vi "Initialise Survey Polygons.vi"(0 "Camera Settings":T2, 5 "Altitude (m)":dbl, 7 "Overlap (%)":dbl, 11 "Error In":errorcluster) -> (2 "Points of Polygon":T1[](array[typedef]) {"Latitude" format="%#_10g"; "Longitude" format="%#_10g"}, 3 "Diameter (km)":dbl, 4 "Start Point":T1 {"Latitude" format="%#_10g"; "Longitude" format="%#_10g"}, 6 "Image Width (m)":dbl, 8 "Image Height (m)":dbl, 10 "Overlap Adjustment (0-1)":dbl, 15 "Error Out":errorcluster)   [LabVIEW 2014]
uses:
  Settings File/Controls/Camera Settings.ctl
  Lat Long Conversion/Controls/PointLatLon.ctl
  Reference/SubVI/Main Map Control Refernce.vi
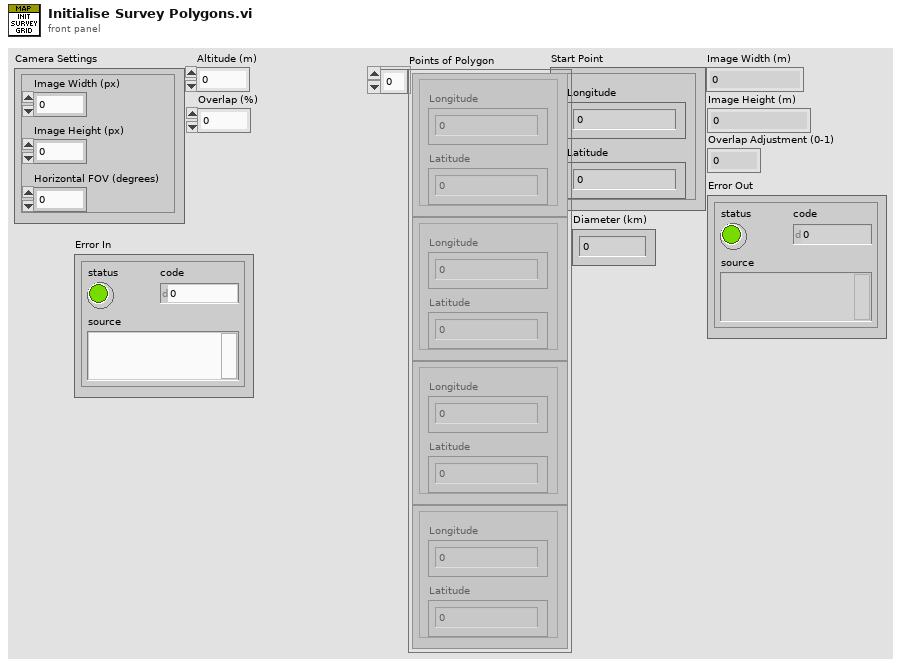
[diagram p1: front panel]
types:
  T1 = typedef "PointLatLon.ctl" = cluster{"Longitude":dbl, "Latitude":dbl}
  T2 = typedef "Camera Settings.ctl" = cluster{"Image Width (px)":dbl, "Image Height (px)":dbl, "Horizontal FOV (degrees)":dbl}
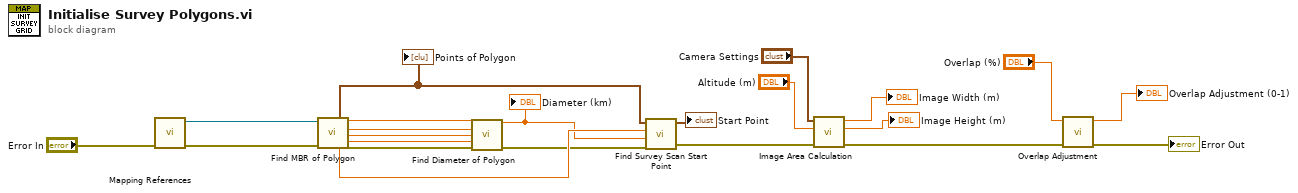
[diagram p0: block diagram]
diagram:
  n1 = call-poly "Mapping References.vi"("Error In"="Error In") -> ("Error Out"=w21:errorcluster, "Main Map Reference"=w22:refnum<k24>)  [unwired: 9 in]
  n2 = call "Find MBR of Polygon.vi"("Overlay Ref"=w22, "error in (no error)"=w21) -> ("Points of Polygon"=w14:T1[], "Min Lat"=w19:dbl, "Min Lon"=w18:dbl, "Max Lat"=w17:dbl, "Max Lon"=w16:dbl, "Bearing Between First two Points"=w13:dbl, "error out"=w15:errorcluster)  [unwired: 7 in]
  "Points of Polygon" <- w14
  n3 = call "Find Diameter of Polygon.vi"("Min Lat"=w19, "Min Lon"=w18, "Max Lat"=w17, "Max Lon"=w16, "Error In"=w15) -> ("Distance (km)"=w12:dbl, "Error Out"=w11:errorcluster)  [unwired: 9 in]
  "Diameter (km)" <- w12
  n4 = call "Find Survey Scan Start Point.vi"("Error In"=w11, "Polygon Diameter (km)"=w12, "Bearing"=w13, "Points of Polygon"=w14) -> ("Error Out"=w10:errorcluster, "Start Point"=→"Start Point":T1)  [unwired: 3 in, 2 out]
  n5 = call "Image Area Calculation.vi"("Error In"=w10, "Altitude (m)"="Altitude (m)", "Camera Settings"="Camera Settings") -> ("Error Out"=w4:errorcluster, "Height (m)"=→"Image Height (m)":dbl, "Width (m)"=→"Image Width (m)":dbl)  [unwired: 5 in, 1 out]
  n6 = call "Overlap Adjustment.vi"("Error In"=w4, "Overlap (%)"="Overlap (%)") -> ("Error Out"=→"Error Out":errorcluster, "Overlap Adjustment (0-1)"=→"Overlap Adjustment (0-1)":dbl)  [unwired: 8 in]
